vi "Dialog Loop settings.vi"(1 "Action(GET)":enum16{"GET", "SET"}(ring), 7 "Anything in":variant, 11 "error in (no error)":errorcluster) -> (8 "Anything out":variant, 10 "Changed since last read":bool, 15 "error out":errorcluster)   [LabVIEW 2010]
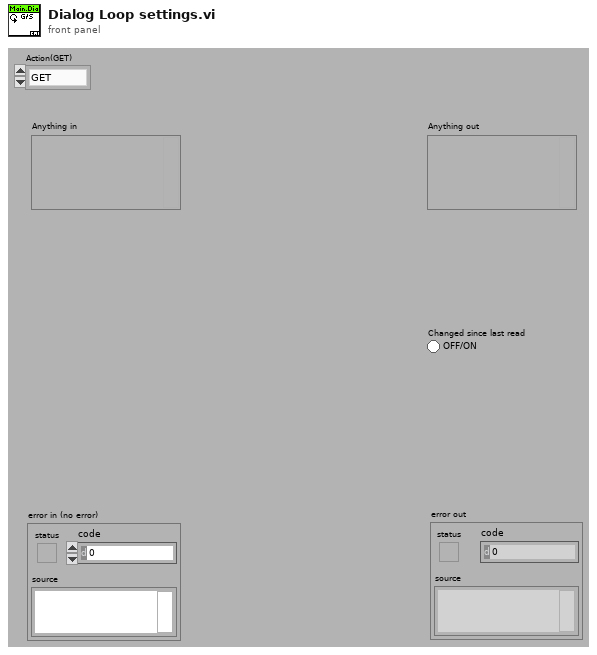
[diagram p1: front panel]
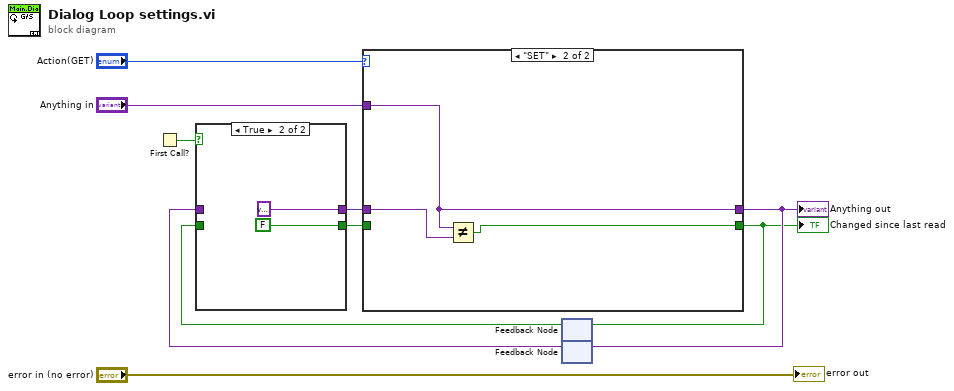
[diagram p0: block diagram]
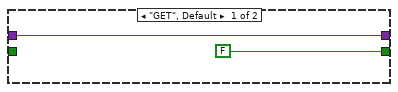
[diagram p3: hidden frame]
diagram:
  n1 = First Call?() -> (First Call?: T/F=w7:bool)
  n2 = feedback #1() -> (w1:bool)  [unwired: 1 in]
  n3 = feedback #2() -> (w8:variant)  [unwired: 1 in]
  n4 = case shown="True" w7 {
    tunnel: w8 -> [w12 _]
    tunnel: [w12 variant ("Anything")] -> w5
    tunnel: [w11 FALSE] -> w2
    tunnel: w1 -> [w11 _]
    frame False {
    }
    frame True {
    }
  }
  n5 = case shown="\"SET\"" "Action(GET)" {
    tunnel: [w16 w19] -> w6
    tunnel: w5 -> [w16 w18]
    tunnel: "Anything in" -> [_ w19]
    tunnel: [FALSE w17] -> w3
    tunnel: w2 -> [_ _]
    frame "GET", Default {
    }
    frame "SET" {
      n6 = Not Equal?(x=w19, y=w18) -> (x != y?=w17:bool)
    }
  }
  "Anything out" <- w6
  "Changed since last read" <- w3
  n7 = feedback-in #1(w3) -> ()
  n8 = feedback-in #2(w6) -> ()
  "error out" <- "error in (no error)"
